vi "GetImage.vi"(2 "error in (no error)":errorcluster, 3 "Time out":i32, 4 "IGxStream":refnum<k24>) -> (0 "error out":errorcluster, 1 "IImageData":refnum<k24>)   [LabVIEW 2013, in "GxLVlib.lvlib"]
uses:
  GxLVlib.lvlib
  C:/Program Files/Daheng Imaging/GalaxySDK/Samples/LabVIEW SDK/x86/GxLVLib/dll/GxIAPINET.dll
  dll/GxIAPINET.dll
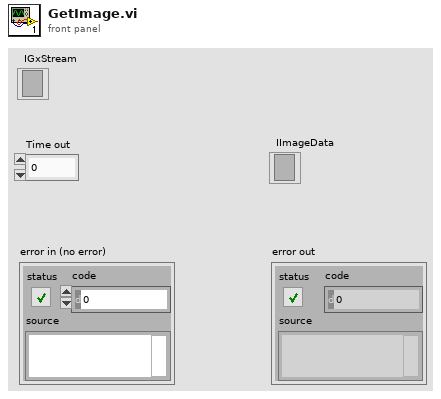
[diagram p1: front panel]
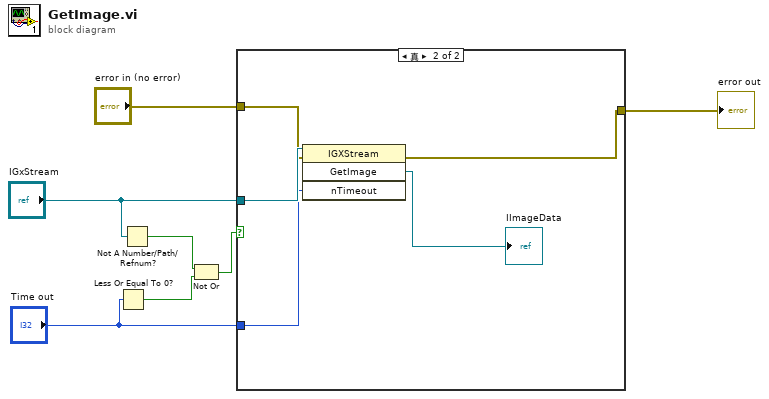
[diagram p0: block diagram]
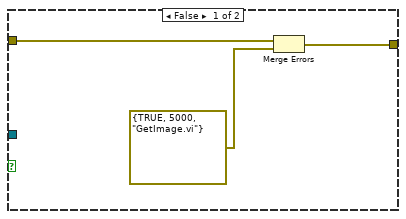
[diagram p2: hidden frame]
diagram:
  n1 = Less Or Equal To 0?(x="Time out") -> (x <= 0?=w6:bool)
  n2 = Not A Number/Path/Refnum?(number/path/refnum="IGxStream") -> (NaN/Path/Refnum?=w7:bool)
  n3 = Not Or(1:w6, 2:w7) -> (0:w5:bool)
  n4 = case shown="真" w5 {
    tunnel: "IGxStream" -> [_ w15]
    tunnel: "Time out" -> [_ w14]
    tunnel: "error in (no error)" -> [w10 w13]
    tunnel: [w8 w12] -> w1
    frame False {
      n5 = Merge Errors(w10, errorcluster {TRUE, 5000, "GetImage.vi"}) -> (w8:errorcluster)
    }
    frame True {
      n6 = invoke class="IGXStream" method="GetImage"(reference=w15, error in=w13, "nTimeout"=w14) -> (error out=w12:errorcluster, "GetImage"=→"IImageData":refnum<k24>)  [unwired: 1 in, 2 out]
    }
  }
  "error out" <- w1
